vi "test_Add Command_Invalid Command or Response Ref Error.vi"(8 "error in (no error)":errorcluster, 11 "TestCase in":refnum<class "Instrument Addon Scripting API Messages Unit Tests.lvclass">) -> (0 "error out":errorcluster, 3 "TestCase out":refnum<class "Instrument Addon Scripting API Messages Unit Tests.lvclass">)   [LabVIEW 2018, in "Instrument Addon Scripting API Messages Unit Tests.lvclass"]
uses:
  Instrument Addon Scripting API Messages Unit Tests.lvclass
  APIs/Scripting API/TypeDefs/Command Settings.ctl
  <vilib>/NI Veristand/Custom Device API/Custom Device Item Ref.ctl
  APIs/Scripting API/TypeDefs/Padding.ctl
  Instrument Addon Scripting API Messages Unit Tests.lvclass/Instrument Addon Scripting API Messages Unit Tests.ctl
  Addon/Addon Shared/SubVIs/Constants.vi
  <vilib>/NI/NI VeriStand Advanced SysDef API/_SubVIs/SysDef.Search.GUID.vi
  <vilib>/addons/_JKI Toolkits/VI Tester/TestCase.llb/TestCase.lvclass
  Instrument Addon Scripting API Test Assets/Instrument Addon Scripting API Test Assets.lvclass
  APIs/Scripting API/Instrument Addon Scripting API.lvlib
  <vilib>/NI Veristand/Custom Device API/Custom Device API.lvlib
  Addon/Addon Shared/Instrument Addon Shared.lvlib
  <vilib>/NI/NI VeriStand Advanced SysDef API/SysDef API/Advanced System Definition.lvlib
  C:/Program Files (x86)/National Instruments/LabVIEW 2018/vi.lib/addons/_JKI Toolkits/VI Tester/TestCase.llb/TestCase.lvclass
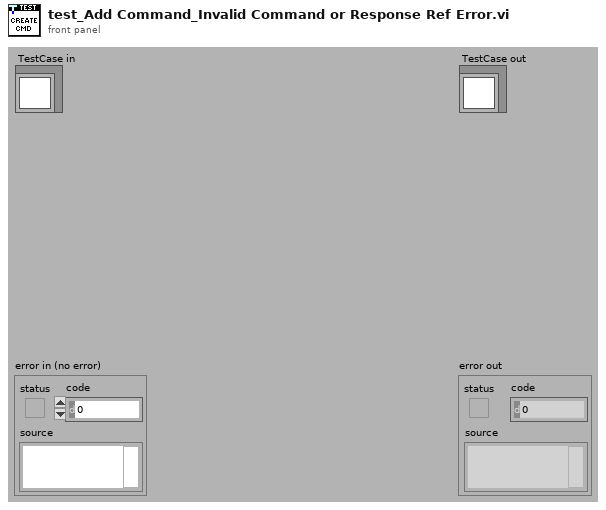
[diagram p1: front panel]
types:
  T1 = typedef "Custom Device API.lvlib/Custom Device Item Ref.ctl" = u64
  T2 = cluster{"Variable Name":string, "Channel Ref in":T1}[]
  T3 = typedef "Instrument Addon Scripting API.lvlib/Command Settings.ctl" = cluster{"Command Format":string, "Linked Channels":cluster{"Variable Name":string, "Channel Ref in":T1}[], "Use Padding?":bool, "Padding":T4}
  T4 = typedef "Instrument Addon Scripting API.lvlib/Padding.ctl" = cluster{"Pad Value":u8, "Length":u32}
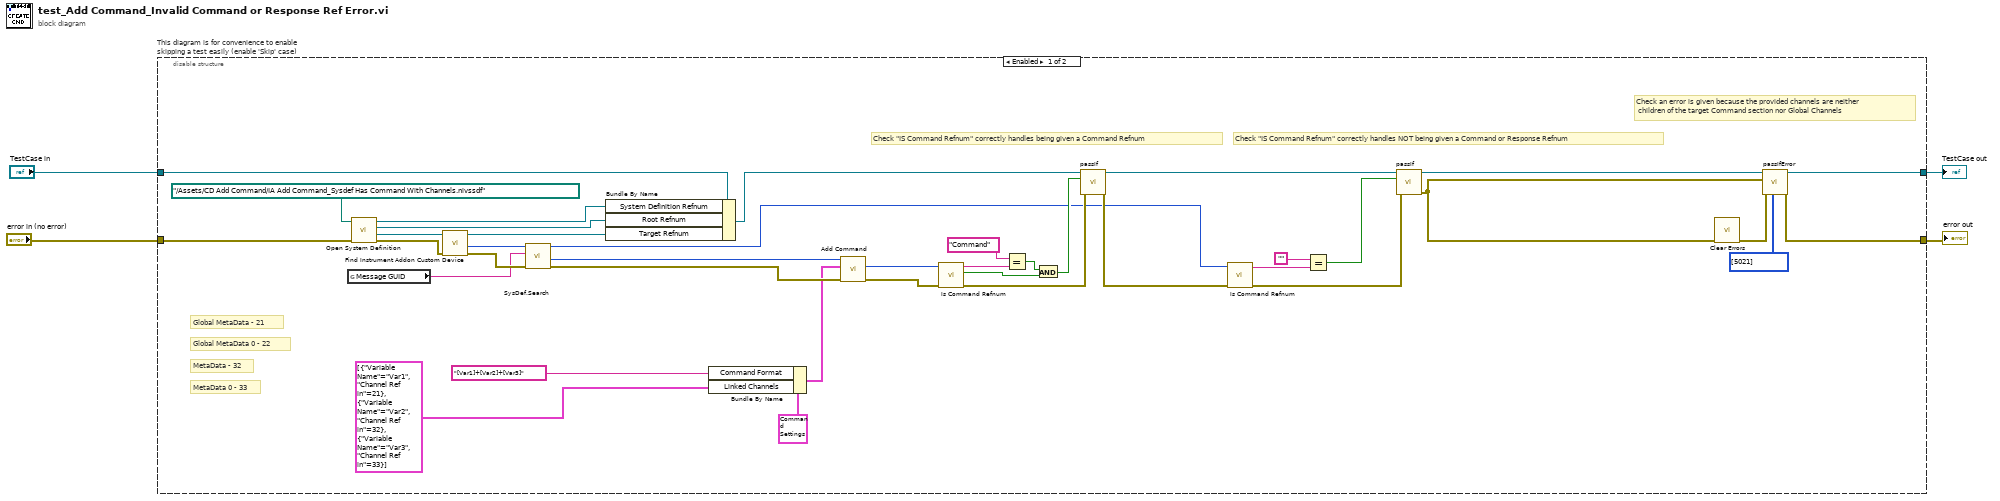
[diagram p0: block diagram]
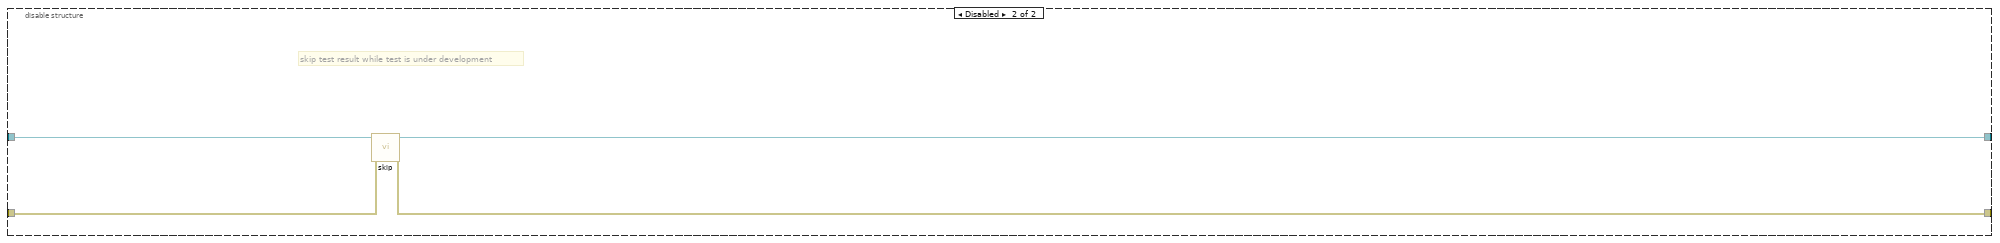
[diagram p2: hidden frame]
diagram:
  n1 = disable-structure "This diagram is for convenience to enable skipping a test easily (enable 'Skip' case)" shown="Enabled" {
    disable-tunnel: "TestCase in" -> [w9 w47]
    disable-tunnel: [w40 w45] -> w1
    disable-tunnel: [w41 w46] -> w3
    disable-tunnel: "error in (no error)" -> [w42 w44]
    frame Enabled {
      # "Check \"IS Command Refnum\" correctly handles NOT being given a Command or Response Refnum"
      # "Check \"IS Command Refnum\" correctly handles being given a Command Refnum"
      # "Check an error is given because the provided channels are neither\n children of the target Command section nor Global Channels"
      # "MetaData 0 - 33"
      # "MetaData - 32"
      # "Global MetaData 0 - 22"
      # "Global MetaData - 21"
      n2 = global read "Constants.vi" "Message GUID"() -> (w36:string)
      n3 = call "Open System Definition.vi"("error in (no error)"=w42, "System Definition File"=path "../Assets/CD Add Command/IA Add Command_Sysdef Has Command With Channels.nivssdf" ("SDF file")) -> ("error out"=w38:errorcluster, "Target Refnum"=w39:refnum<k24>, "Root Refnum"=w6:refnum<k24>, "System Definition Refnum"=w7:refnum<k24>)  [unwired: 6 in]
      n4 = call "Find Instrument Addon Custom Device.vi"("error in"=w38, "target in"=w39) -> ("error out"=w37:errorcluster, "NodeID"=w31:u64, "target out"=w5:refnum<k24>)  [unwired: 7 in]
      n5 = call-poly <vilib>:"SysDef.Search.vi"("error in (no error)"=w37, "GUID"=w36, "nodeID"=w31) -> ("error out"=w35:errorcluster, "Value out"=w27:u64, "nodeID out"=w17:u64)  [unwired: 5 in, 1 out]
      n6 = Bundle By Name(cluster=w9, "System Definition Refnum"=w7, "Root Refnum"=w6, "Target Refnum"=w5) -> (w8:refnum<class "Instrument Addon Scripting API Messages Unit Tests.lvclass">)
      n7 = Bundle By Name(cluster=T3 {"Command Format"="[Var1]+[Var2]", "Linked Channels"=[{"Variable Name"="Var1", "Channel Ref in"=32}, {"Variable Name"="Var2", "Channel Ref in"=33}], "Use Padding?"=FALSE, "Padding"={"Pad Value"=0, "Length"=0}} ("Settings"), "Command Format"="[Var1]+[Var2]+[Var3]", "Linked Channels"=T2 [{"Variable Name"="Var1", "Channel Ref in"=21}, {"Variable Name"="Var2", "Channel Ref in"=32}, {"Variable Name"="Var3", "Channel Ref in"=33}]) -> (w33:T3)
      n8 = call "Add Command.vi"("Error In"=w35, "Settings"=w33, "Message Refnum In"=w27) -> ("Error Out"=w25:errorcluster, "Command Refnum"=w26:T1)  [unwired: 6 in, 1 out]
      n9 = call "Is Command Refnum.vi"("error in (no error)"=w25, "Command/Response Refnum in"=w26) -> ("error out"=w24:errorcluster, "Is Command?"=w20:bool, "Command/Response out"=w23:string)  [unwired: 7 in]
      n10 = Equal?(x="Command", y=w23) -> (x = y?=w21:bool)
      n11 = And(x=w21, y=w20) -> (x .and. y?=w19:bool)
      n12 = call-dynamic "passIf.vi"("error in (no error)"=w24, "pass"=w19, "TestCase in"=w8) -> ("error out"=w18:errorcluster, "TestCase out"=w11:refnum<class "Instrument Addon Scripting API Messages Unit Tests.lvclass">)  [unwired: 7 in]
      n13 = call "Is Command Refnum.vi"("error in (no error)"=w18, "Command/Response Refnum in"=w17) -> ("error out"=w13:errorcluster, "Command/Response out"=w15:string)  [unwired: 7 in, 1 out]
      n14 = Equal?(x="", y=w15) -> (x = y?=w14:bool)
      n15 = call-dynamic "passIf.vi"("error in (no error)"=w13, "pass"=w14, "TestCase in"=w11) -> ("error out"=w12:errorcluster, "TestCase out"=w10:refnum<class "Instrument Addon Scripting API Messages Unit Tests.lvclass">)  [unwired: 7 in]
      n16 = call <vilib>:"Clear Errors.vi"("error in (no error)"=w12) -> ("error out"=w29:errorcluster)  [unwired: 5 in, 1 out]
      n17 = call-dynamic "passIfError.vi"("passing error codes (default = any error code)"=i32[] [5021], "error in (no error)"=w29, "error"=w12, "TestCase in"=w10) -> ("error out"=w41:errorcluster, "TestCase out"=w40:refnum<class "Instrument Addon Scripting API Messages Unit Tests.lvclass">)  [unwired: 6 in]
    }
    frame Disabled {
      # "skip test result while test is under development"
      n18 = call <vilib>:"skip.vi"("error in (no error)"=w44, "TestCase in"=w47) -> ("error out"=w46:errorcluster, "TestCase out"=w45:refnum<class "Instrument Addon Scripting API Messages Unit Tests.lvclass">)  [unwired: 8 in]
    }
  }
  "error out" <- w3
  "TestCase out" <- w1
